vi "Network_Get_Shared_Variables_v4.vi"(2 "error in (no error)":errorcluster, 3 "Source of Data":refnum<k21>) -> (0 "error out":errorcluster, 1 "Igor Instruction String":string[](array[string]))   [LabVIEW 2015]
doc: "Uses DataSocket technology to read live images."
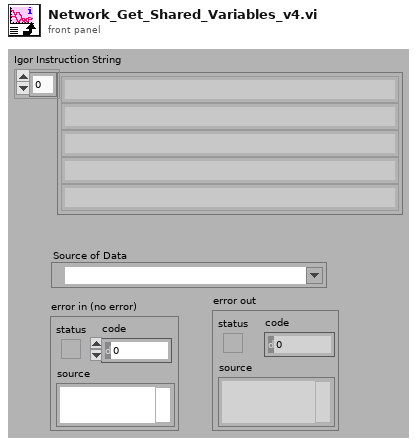
[diagram p1: front panel]
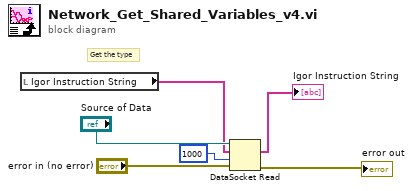
[diagram p0: block diagram]
diagram:
  # "Get the type"
  n1 = local read "Igor Instruction String"() -> (w2:string[])
  n2 = DataSocket Read(8:"error in (no error)", 9:1000 ("ms timeout (10000)"), 10:w2, 11:"Source of Data") -> (0:→"error out":errorcluster, 2:→"Igor Instruction String":string[])  [unwired: 6 out]
